vi "Find Project Files With Issues.vi"() -> (0 "error out":errorcluster, 2 "Pass":bool)   [LabVIEW 2015, in "Sequencer Module tests.lvlib"]
uses:
  Sequencer Module tests.lvlib
  <vilib>/regexp/Match Regular Expression.xnode
panel:
  out "Items With Conflicts":string[](array[string])
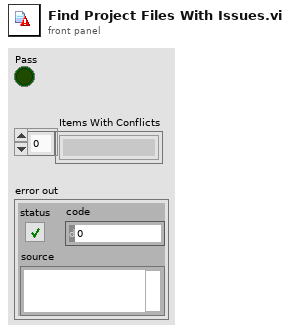
[diagram p1: front panel]
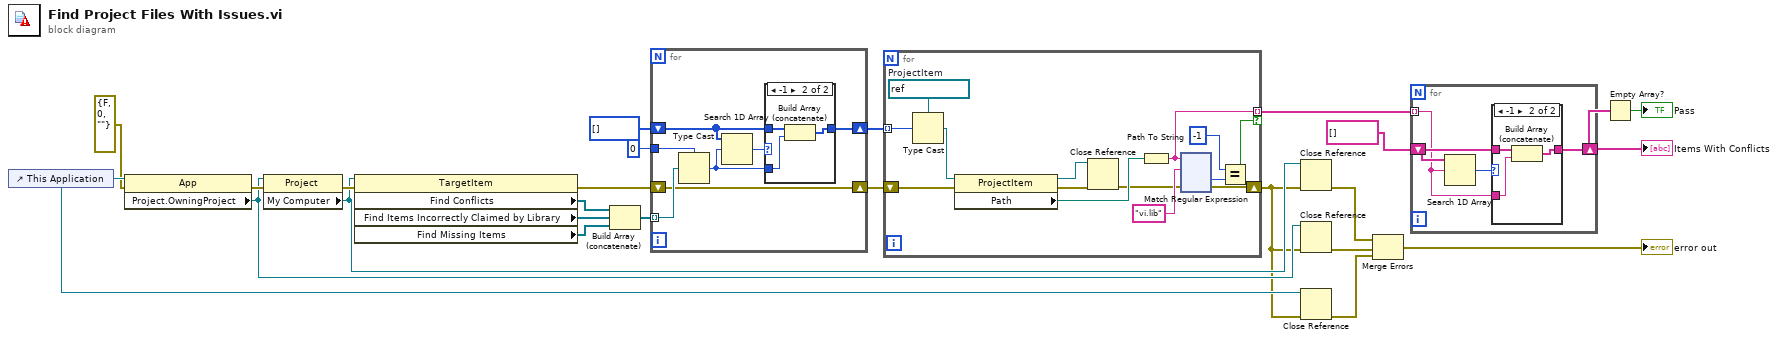
[diagram p0: block diagram]
diagram:
  n1 = control-ref of="This Application"() -> (w12:refnum<vi>)
  n2 = property class="App"(reference=w12, error in=errorcluster {"status"=FALSE, "code"=0, "source"=""} ("error in (no error)")) -> (error out=w18:errorcluster, "Project.OwningProject"=w13:refnum<vi>)  [unwired: 1 out]
  n3 = property class="Project"(reference=w13, error in=w18) -> (error out=w17:errorcluster, "My Computer"=w14:refnum<vi>)  [unwired: 1 out]
  n4 = property class="TargetItem"(reference=w14, error in=w17) -> (error out=w16:errorcluster, "Find Conflicts"=w24:refnum<vi>[], "Find Items Incorrectly Claimed by Library"=w11:refnum<vi>[], "Find Missing Items"=w23:refnum<vi>[])  [unwired: 1 out]
  n5 = Build Array (concatenate)(w24, w11, w23) -> (w22:refnum<vi>[])
  n6 = for {
    tunnel: w22 -> [w31] mode=indexing
    shift-right: [w26] -> w19
    shift-left: u32[] [] ("appended array") -> [w28]
    tunnel: u32 0 -> [w30]
    shift-right: [w25] -> w15
    shift-left: w16 -> [w25]
    n7 = Type Cast(type=w30, x=w31) -> (*(type *) &x=w27:u32)
    n8 = Search 1D Array(1D array=w28, element=w27) -> (index of element=w29:i32)  [unwired: 1 in]
    n9 = case shown="-1" w29 {
      tunnel: w28 -> [w32 w35]
      tunnel: w27 -> [_ w34]
      tunnel: [w32 w33] -> w26
      frame 0, Default {
      }
      frame -1 {
        n10 = Build Array (concatenate)(w35, w34) -> (w33:u32[])
      }
    }
  }
  n11 = for {
    tunnel: w19 -> [w49] mode=indexing
    shift-right: [w37] -> w5
    shift-left: w15 -> [w46]
    tunnel: [w44] -> w9 mode=indexing if=w36
    w48 = refnum<vi> refnum  # ProjectItem
    n12 = Type Cast(type=w48, x=w49) -> (*(type *) &x=w47:refnum<vi>)
    n13 = property class="ProjectItem"(reference=w47, error in=w46) -> (reference out=w40:refnum<vi>, error out=w39:errorcluster, "Path"=w45:path)
    n14 = Close Reference(reference=w40, error in (no error)=w39) -> (error out=w38:errorcluster)
    n15 = Path To String(path=w45) -> (string=w44:string)
    n16 = xnode "Match Regular Expression"("input string"=w44, "regular expression"="vi.lib", "error in"=w38) -> ("offset past match"=w42:i32, "error out"=w37:errorcluster)  [unwired: 3 in, 3 out]
    n17 = Equal?(x=-1 ("y"), y=w42) -> (x = y?=w36:bool)
  }
  n18 = Close Reference(reference=w14, error in (no error)=w5) -> (error out=w4:errorcluster)
  n19 = Close Reference(reference=w13, error in (no error)=w5) -> (error out=w3:errorcluster)
  n20 = Close Reference(reference=w12, error in (no error)=w5) -> (error out=w2:errorcluster)
  n21 = Merge Errors(w4, w3, w2) -> (→"error out":errorcluster)
  n22 = for {
    tunnel: w9 -> [w165] mode=indexing
    shift-right: [w164] -> w7
    shift-left: string[] [] -> [w166]
    n23 = Search 1D Array(1D array=w166, element=w165) -> (index of element=w167:i32)  [unwired: 1 in]
    n24 = case shown="-1" w167 {
      tunnel: w166 -> [w168 w171]
      tunnel: [w168 w170] -> w164
      tunnel: w165 -> [_ w169]
      frame 0, Default {
      }
      frame -1 {
        n25 = Build Array (concatenate)(w171, w169) -> (w170:string[])
      }
    }
  }
  "Items With Conflicts" <- w7
  n26 = Empty Array?(array=w7) -> (empty?=→"Pass":bool)
